vi "Global_ACT_Data Out.vi"() -> ()   [LabVIEW 2023, in "Feeder_ACT.lvlib"]
uses:
  Feeder_ACT.lvlib
  ENUM_ACT_State.ctl
panel:
  in  "Feeder State":T1
  out "ACT_Feeder_PusherBack":bool
  in  "ACT_Feeder_Pusher Position Set":dbl
  in  "ACT_Feeder_CycleTime(S)":dbl
  in  "ACT_Feeder_Puller Speed":dbl
  # "The Names of the Data items in the Global Variable MUST describe who the Single Writer is\nFor Actuator Globals the the naming convention is\n   \nACT_Lib Name_Data Name\n\nExamples:\nACT_Drive_X axis\nACT_Hopper_AgitatorSpeed"
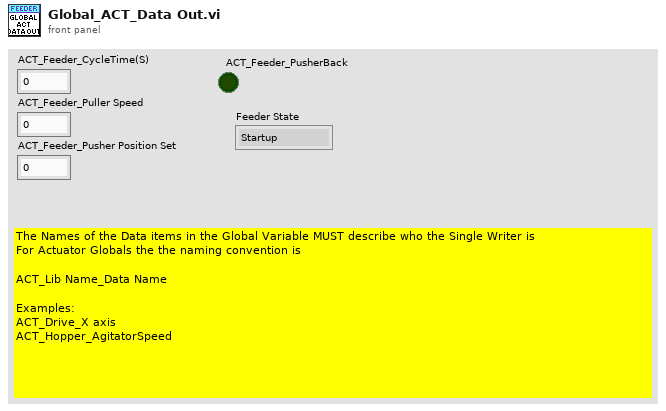
[diagram p1: front panel]
types:
  T1 = typedef "Feeder_ACT.lvlib/ENUM_ACT_State.ctl" = enum16{"Startup", "Back Waiting", "Push Feeding", "Retracting", "Shutdown"}
diagram:
